vi "fetch_and_translate_trigger.vi"(8 "error in (no error)":errorcluster, 11 "StageDL090409Scaffold in":refnum<class "StageDL090409Scaffold.lvclass">) -> (0 "error out":errorcluster, 1 "sender TLC type":T1=enum."ImagingMode", 2 "statechart trigger":T2, 3 "StageDL090409Scaffold out":refnum<class "StageDL090409Scaffold.lvclass">)   [LabVIEW 2010, in "StageDL090409Scaffold.lvclass"]
uses:
  StageDL090409Scaffold.lvclass
  internal_trigger_enum.ctl
  common/enumerations/top-level_component_type_enum.ctl
  GenericStage/GenericStage/trigger_enum.ctl
  GenericStage/GenericStage/GenericStage.lvclass
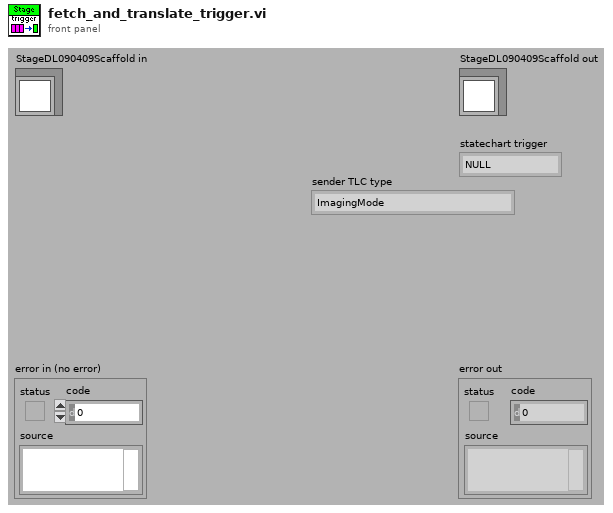
[diagram p1: front panel]
types:
  T1 = typedef "top-level_component_type_enum.ctl" = enum16{"undefined", "ImagingMode", "ScanHead", "DAQ", "ImageAssembler", "Display", "DataCollection", "Analyser", "Stimulator", "ExperimentController", "Instrument", "Stage"}
  T2 = typedef "StageDL090409Scaffold.lvclass/internal_trigger_enum.ctl" = enum16{"NULL", "initialise", "terminate", "move", "update position", "set origin", "return to origin", "attach observer", "detach observer"}
  T3 = typedef "GenericStage.lvclass/trigger_enum.ctl" = enum16{"NULL", "move", "update position", "set origin", "return to origin"}
  T4 = typedef "GenericToplevelComponent.lvclass/common_trigger_enum.ctl" = enum16{"NULL", "initialise", "terminate", "fetch command", "fetch data", "attach observer", "register as observer", "detach observer", "acknowledge", "start", "stop", "sweep started", "sweep finished", "experiment started", "experiment stopped"}
  T5 = typedef "trigger_type_enum.ctl" = enum8{"external", "internal", "common"}
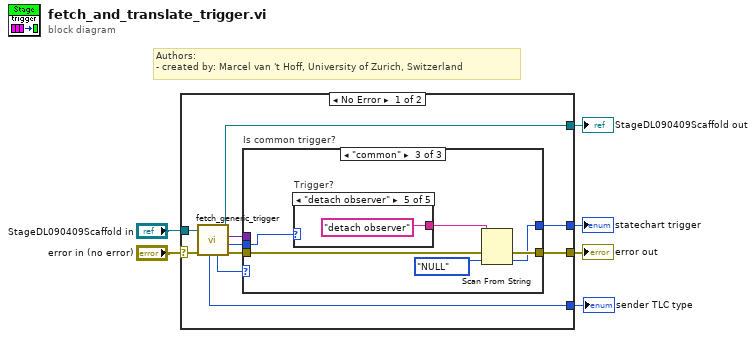
[diagram p0: block diagram]
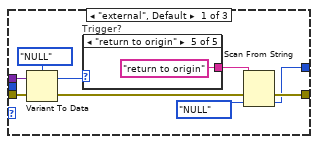
[diagram p2: hidden frame]
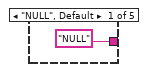
[diagram p3: hidden frame]
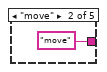
[diagram p4: hidden frame]
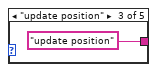
[diagram p5: hidden frame]
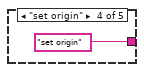
[diagram p6: hidden frame]
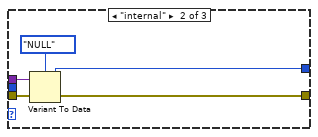
[diagram p7: hidden frame]
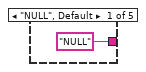
[diagram p8: hidden frame]
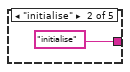
[diagram p9: hidden frame]
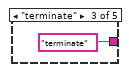
[diagram p10: hidden frame]
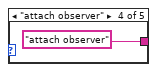
[diagram p11: hidden frame]
diagram:
  # "Authors: \n- created by: Marcel van 't Hoff, University of Zurich, Switzerland"
  n1 = case shown="No Error" "error in (no error)" {
    selector: "error in (no error)" -> [w13 w48]
    tunnel: [w11 w48] -> w5
    tunnel: [w14 w47] -> w3
    tunnel: "StageDL090409Scaffold in" -> [w15 w47]
    tunnel: [w16 _] -> w1
    tunnel: [w7 _] -> w2
    frame No Error {
      n2 = call-dynamic "fetch_generic_trigger.vi"("error in (no error)"=w13, "GenericToplevelComponent in"=w15) -> ("error out"=w12:errorcluster, "common trigger"=w8:T4, "trigger"=w10:variant, "GenericToplevelComponent out"=w14:refnum<class "StageDL090409Scaffold.lvclass">, "trigger type"=w9:T5, "sender TLC type"=w7:T1)  [unwired: 3 in, 1 out]
      n3 = case "Is common trigger?" shown="\"common\"" w9 {
        tunnel: [w18 w32 w37] -> w16
        tunnel: w12 -> [w24 w34 w40]
        tunnel: [w20 w33 w39] -> w11
        tunnel: w10 -> [w23 w35 _]
        tunnel: w8 -> [_ _ w41]
        frame "external", Default {
          n4 = Variant To Data(error in=w24, Variant=w23, type=trigger_enum."NULL" ("trigger")) -> (error out=w21:errorcluster, data=w25:T3)
          n5 = case "Trigger?" shown="\"return to origin\"" w25 {
            tunnel: ["NULL" "move" "update position" "set origin" "return to origin"] -> w19
            frame "NULL", Default {
            }
            frame "move" {
            }
            frame "update position" {
            }
            frame "set origin" {
            }
            frame "return to origin" {
            }
          }
          n6 = Scan From String(input string=w19, error in=w21, default 1=internal_trigger_enum."NULL" ("statechart trigger")) -> (error out=w20:errorcluster, output 1=w18:T2)  [unwired: 2 in, 2 out]
        }
        frame "internal" {
          n7 = Variant To Data(error in=w34, Variant=w35, type=internal_trigger_enum."NULL" ("statechart trigger")) -> (error out=w33:errorcluster, data=w32:T2)
        }
        frame "common" {
          n8 = case "Trigger?" shown="\"detach observer\"" w41 {
            tunnel: ["NULL" "initialise" "terminate" "attach observer" "detach observer"] -> w36
            frame "NULL", Default {
            }
            frame "initialise" {
            }
            frame "terminate" {
            }
            frame "attach observer" {
            }
            frame "detach observer" {
            }
          }
          n9 = Scan From String(input string=w36, error in=w40, default 1=internal_trigger_enum."NULL" ("statechart trigger")) -> (error out=w39:errorcluster, output 1=w37:T2)  [unwired: 2 in, 2 out]
        }
      }
    }
    frame Error {
    }
  }
  "error out" <- w5
  "StageDL090409Scaffold out" <- w3
  "statechart trigger" <- w1
  "sender TLC type" <- w2
